vi "WTIME lookup table.vi"(10 "Incoming Data in":u8[](array[numeric])) -> (2 "WAIT TIME (s)":dbl)   [LabVIEW 2016, in "AMS TS3472 Light Sensor.lvlib" / "AMS TCS3472.lvclass"]
uses:
  AMS TCS3472.lvclass
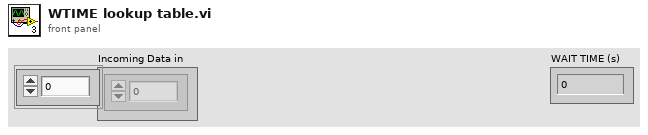
[diagram p1: front panel]
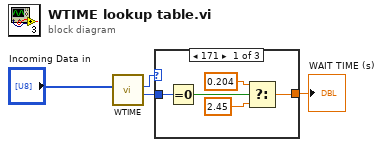
[diagram p0: block diagram]
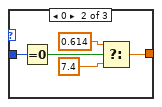
[diagram p2: hidden frame]
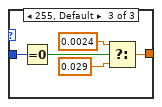
[diagram p3: hidden frame]
diagram:
  n1 = call "WTIME.vi"("Incoming Data in"="Incoming Data in") -> ("CONFIG"=w2:u8, "WTIME"=w3:u8)  [unwired: 9 in]
  n2 = case shown="171" w3 {
    tunnel: [w5 w11 w15] -> w1
    tunnel: w2 -> [w6 w14 w16]
    frame 171 {
      n3 = Equal To 0?(x=w6) -> (x = 0?=w9:bool)
      n4 = Select(t=0.204, s=w9, f=2.45) -> (s? t:f=w5:dbl)
    }
    frame 0 {
      n5 = Equal To 0?(x=w14) -> (x = 0?=w13:bool)
      n6 = Select(t=0.614, s=w13, f=7.4) -> (s? t:f=w11:dbl)
    }
    frame 255, Default {
      n7 = Equal To 0?(x=w16) -> (x = 0?=w19:bool)
      n8 = Select(t=0.0024, s=w19, f=0.029) -> (s? t:f=w15:dbl)
    }
  }
  "WAIT TIME (s)" <- w1
